vi "Load Hardware.vi"(8 "error in (no error)":errorcluster, 10 "Program only changes":bool, 11 "Pulseblaster in":refnum<class "Slave_Pulseblaster.lvclass">) -> (0 "error out":errorcluster, 3 "Pulseblaster out":refnum<class "Slave_Pulseblaster.lvclass">)   [LabVIEW 2013, in "Slave_Pulseblaster.lvclass"]
doc: "While \"Program only changes\" functionality has been written for the PulseBlaster, it is currently diabled as the Clear Hardware \"PB close\" is throwing an error (I assume without the corresponting \"init\" call from Load Hardware when no changes are made).\n\nThe PulseBlaster will program every time."
uses:
  Slave_Pulseblaster.lvclass
  Slave_Pulseblaster.lvclass/Slave_Pulseblaster.ctl
  Utils/Unequal_safe/Unequal_Safe_VLIWarray.vi
  Utils_devs/SpinAPI/SpinAPI-Interface.lvlib
panel:
  out "Last HWIs":T1(array[cluster])
  out "Program?":bool
  out "Names encountered":string[](array[string])
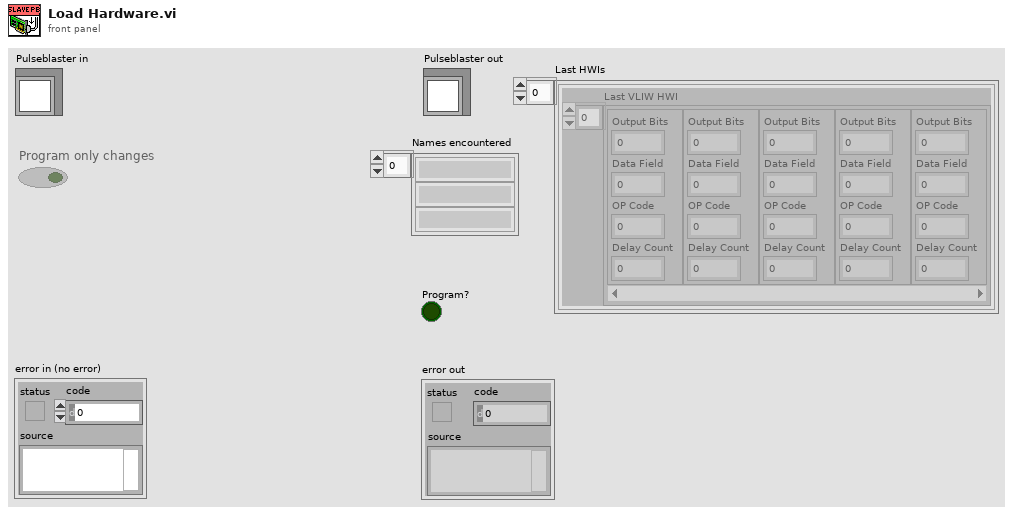
[diagram p1: front panel]
types:
  T1 = cluster{"Last VLIW HWI":cluster{"Output Bits":u32, "Data Field":u32, "OP Code":u8, "Delay Count":u64}[]}[]
  T2 = cluster{"Output Bits":u32, "Data Field":u32, "OP Code":u8, "Delay Count":u64}[]
  T3 = cluster{"Last VLIW HWI":cluster{"Output Bits":u32, "Data Field":u32, "OP Code":u8, "Delay Count":u64}[]}
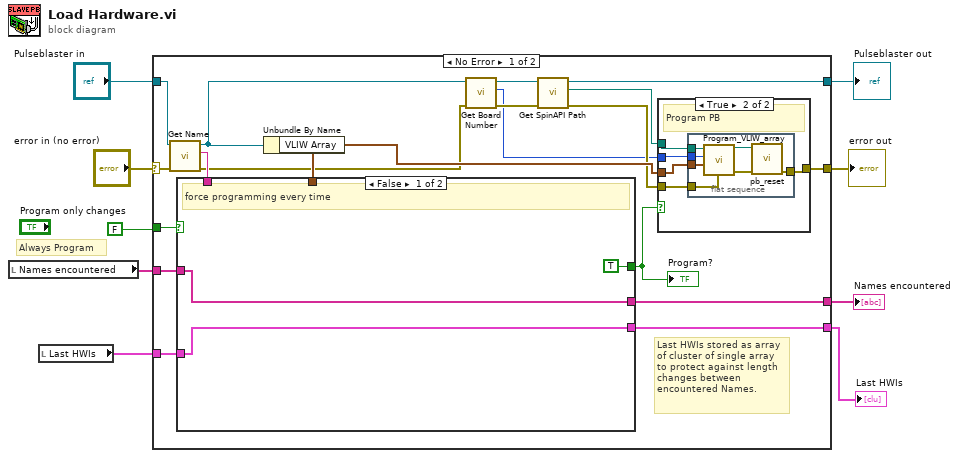
[diagram p0: block diagram]
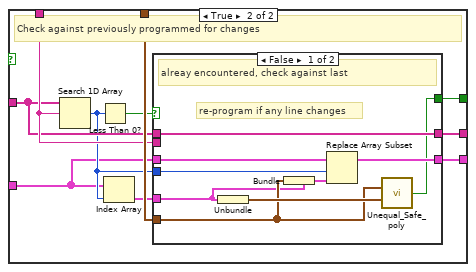
[diagram p2: hidden frame]
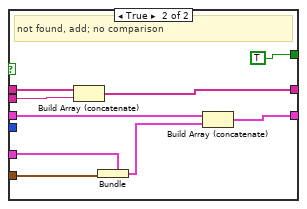
[diagram p3: hidden frame]
diagram:
  # "Always Program"
  n1 = local read "Names encountered"() -> (w4:string[])
  n2 = local read "Last HWIs"() -> (w3:T1)
  n3 = case shown="No Error" "error in (no error)" {
    selector: "error in (no error)" -> [w27 w76]
    tunnel: [w28 w76] -> w6
    tunnel: "Pulseblaster in" -> [w26 w75]
    tunnel: [w12 w75] -> w7
    tunnel: FALSE ("Program only changes") -> [w18 _]
    tunnel: w3 -> [w23 w74]
    tunnel: [w22 w74] -> w2
    tunnel: [w24 w73] -> w5
    tunnel: w4 -> [w19 w73]
    frame No Error {
      # "Last HWIs stored as array\nof cluster of single array\nto protect against length\nchanges between\nencountered Names."
      n4 = call-dynamic "Get Name.vi"("error in (no error)"=w27, "Device in"=w26) -> ("error out"=w16:errorcluster, "Name"=w20:string, "Device out"=w17:refnum<class "Slave_Pulseblaster.lvclass">)  [unwired: 7 in]
      n5 = Unbundle By Name(w17) -> ("VLIW Array"=w21:T2)
      n6 = case shown="False" w18 {
        tunnel: [TRUE ("Diff?") w41] -> w25
        tunnel: [w31 w40] -> w24
        tunnel: w23 -> [w30 w33]
        tunnel: [w30 w39] -> w22
        tunnel: w21 -> [_ w38]
        tunnel: w20 -> [_ w36]
        tunnel: w19 -> [w31 w35]
        frame False {
          # "force programming every time"
        }
        frame True {
          # "Check against previously programmed for changes"
          n7 = Search 1D Array(1D array=w35, element=w36) -> (index of element=w34:i32)  [unwired: 1 in]
          n8 = Less Than 0?(x=w34) -> (x < 0?=w37:bool)
          n9 = Index Array(array=w33, index=w34) -> (element=w32:T3)
          n10 = case shown="False" w37 {
            tunnel: w36 -> [_ w58]
            tunnel: w35 -> [w50 w59]
            tunnel: [w50 w57] -> w40
            tunnel: [w46 TRUE] -> w41
            tunnel: w33 -> [w49 w53]
            tunnel: w38 -> [w43 w54]
            tunnel: w34 -> [w48 _]
            tunnel: [w47 w55] -> w39
            tunnel: w32 -> [w42 w51]
            frame False {
              # "re-program if any line changes"
              # "alreay encountered, check against last"
              n11 = Unbundle(w42) -> ("Last VLIW HWI"=w45:T2)
              n12 = Bundle(cluster=w42, "Last VLIW HWI"=w43) -> (w44:T3)
              n13 = Replace Array Subset(array=w49, new element=w44, index=w48) -> (w47:T1)
              n14 = call-poly "Unequal_Safe_poly.vi"("VLIW Array x"=w43, "VLIW Array y"=w45) -> ("Diff?"=w46:bool)  [unwired: 12 in, 1 out]
            }
            frame True {
              # "not found, add; no comparison"
              n15 = Build Array (concatenate)(w59, w58) -> (w57:string[])
              n16 = Bundle(cluster=w51, "Last VLIW HWI"=w54) -> (w52:T3)
              n17 = Build Array (concatenate)(w53, w52) -> (w55:T1)
            }
          }
        }
      }
      "Program?" <- w25
      n18 = call-dynamic "Get Board Number.vi"("error in (no error)"=w16, "Pulseblaster in"=w17) -> ("error out"=w15:errorcluster, "Board Number"=w10:i32, "Pulseblaster out"=w13:refnum<class "Slave_Pulseblaster.lvclass">)  [unwired: 7 in]
      n19 = call-dynamic "Get SpinAPI Path.vi"("error in (no error)"=w15, "Pulseblaster in"=w13) -> ("error out"=w14:errorcluster, "SpinAPI Path"=w11:path, "Pulseblaster out"=w12:refnum<class "Slave_Pulseblaster.lvclass">)  [unwired: 7 in]
      n20 = case shown="True" w25 {
        tunnel: [w60 w61] -> w28
        tunnel: w14 -> [w60 w65]
        tunnel: w21 -> [_ w64]
        tunnel: w11 -> [_ w62]
        tunnel: w10 -> [_ w63]
        frame False {
          # "No need to program"
        }
        frame True {
          # "Program PB"
          n21 = flat-sequence {
            tunnel: w65 -> [w72]
            tunnel: w64 -> [w71]
            tunnel: w63 -> [w70]
            tunnel: w62 -> [w69]
            tunnel: [w66] -> w61
            frame #0 {
              n22 = call "Program_VLIW_array.vi"("path in"=w69, "board_num"=w70, "PulseBlaster\nVLIW Array"=w71, "error in"=w72) -> ("path out"=w68:path, "error out"=w67:errorcluster)  [unwired: 2 in]
              n23 = call "pb_reset.vi"("error in (no error)"=w67, "path in"=w68) -> ("error out"=w66:errorcluster)  [unwired: 8 in, 1 out]
            }
          }
        }
      }
    }
    frame Error {
    }
  }
  "error out" <- w6
  "Pulseblaster out" <- w7
  "Names encountered" <- w5
  "Last HWIs" <- w2
